vi "Exercise3.vi"() -> ()   [LabVIEW 2016]
uses:
  <vilib>/Utility/file.llb/Write Delimited Spreadsheet (DBL).vi
  Classes/Controller/Motion/Motion Folder/Motion.lvclass
  Classes/Controller/I-O/I-O Folder/I-O.lvclass
  Classes/Controller/Controller Folder/Controller.lvclass
panel:
  in  "file path (dialog if empty)":path=path "D:/Gantry_General/Qualification Results/Exercise3/FInal Combine.txt"
  in  "Final Sensor":path=path "D:/Gantry_General/Qualification Results/Exercise3/Final Sensor.txt"
  out "Bellow position 4":dbl[](array[numeric])=[936.279, 64.123, 66.649, 0.0]
  out "Bellow position 3":dbl[](array[numeric])=[353.0239567258022, 98.85055613080435, 59.0791979543358, 1.5763766432237363]
  out "Bellow position 2":dbl[](array[numeric])=[608.3519774161907, 47.80550407841485, 51.02600004353454, 0.5267134461077569]
  out "Bellow position":dbl[](array[numeric])=[936.279, 64.123, 66.649, 0.0]
  in  "Stop":bool
  in  "Put down pickup tool":bool
  in  "Put down sensor":bool
  in  "Pickup Sensor":bool
  in  "Pickup Pickup Tool":bool
  out "Vacuum OK":bool
  in  "Tray 3":bool
  out "Pickup Tool Center":dbl[](array[numeric])=[1056.142, 74.613, 66.649, 0.0]
  in  "Pickup Tool rotation":dbl=3.14159
  in  "Pickup Tool Path":path=path "D:/Gantry_General/Qualification Results/Exercise3/Pickuptool.txt"
  in  "Sensor":bool
  out "Sensor Center":dbl[](array[numeric])=[728.2149774161908, 58.29550407841485, 51.02600004353454, 0.5267134461077569]
  in  "Sensor rotation":dbl=3.14159
  in  "Sensor Path":path=path "D:/Gantry_General/Qualification Results/Exercise3/Sensor.txt"
  in  "Place position wrt\n Tray Center":dbl[](array[numeric])=[95.0, 0.0, 0.0, 0.0]
  in  "Tray Path":path=path "D:/Gantry_General/Qualification Results/Exercise3/tray.txt"
  in  "Tray rotation":dbl=5.14872
  out "Tray Center":dbl[](array[numeric])=[472.8869567258022, 109.34055613080434, 59.0791979543358, 1.5763766432237363]
  in  "Alignment finish":bool
  in  "Tray":bool
  in  "Final position vacuum":i32=22
  in  "Baseplate mark vacuum":i32=-1
  in  "Sensor Vacuum":i32=20
  in  "Baseplate Region Vacuum":i32=23
  in  "Sensor Regiopn Vacuum":i32=21
  in  "Pickup?":bool=TRUE
  in  "Pickup Go":bool
  # "Gantry Qualification Exercise 3\n1. Place Material"
  # "Alignment settings"
  # "Initialize Vacuum Setup"
  # "( rotation expressed in radians )"
  # "Align material"
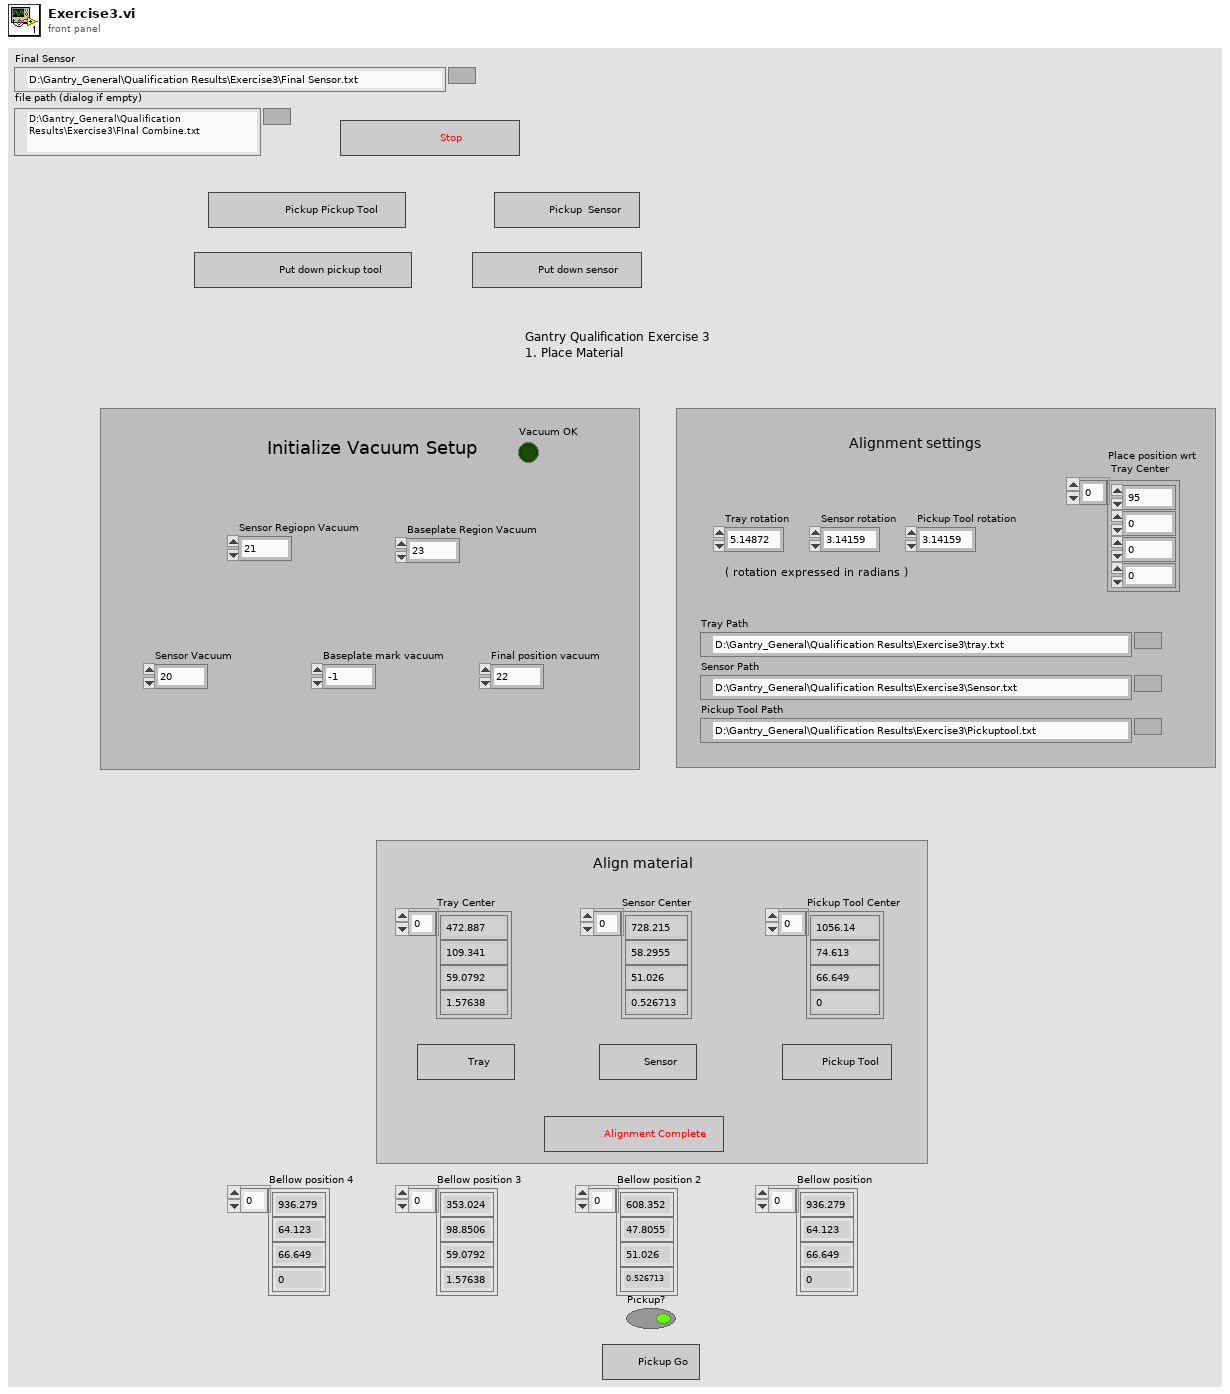
[diagram p1: front panel]
types:
  T1 = typedef "Controller.lvclass/Controllers.ctl" = cluster{"Copy of Motion.lvclass":refnum<class "Motion.lvclass">, "Copy of I-O.lvclass ":refnum<class "I-O.lvclass">, "Copy of Dispenser.lvclass":refnum<class "Dispenser.lvclass">}
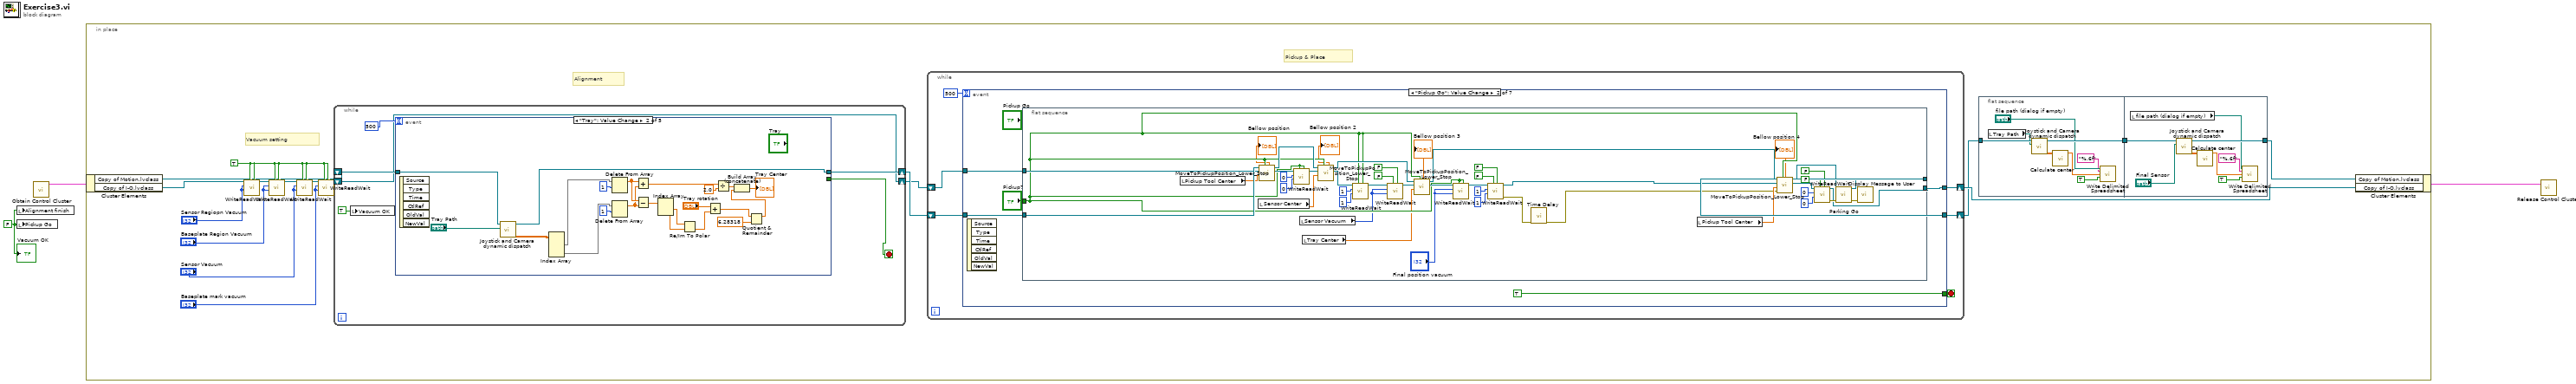
[diagram p0: block diagram]
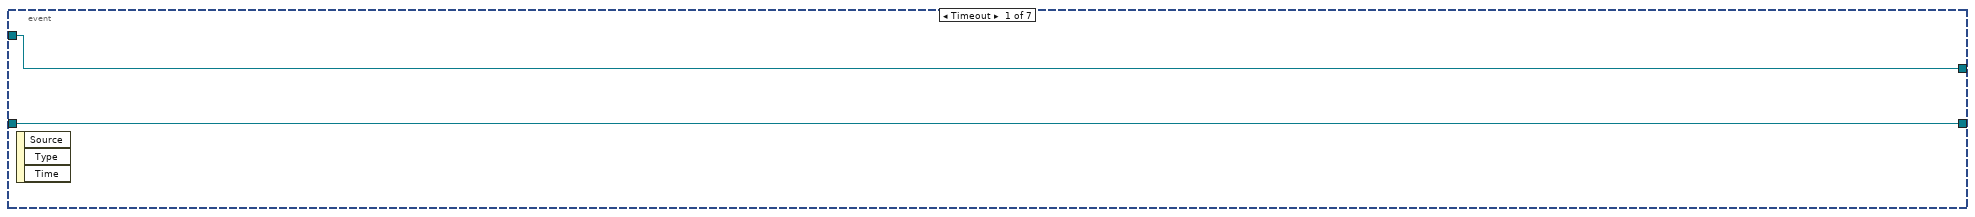
[diagram p2: hidden frame]
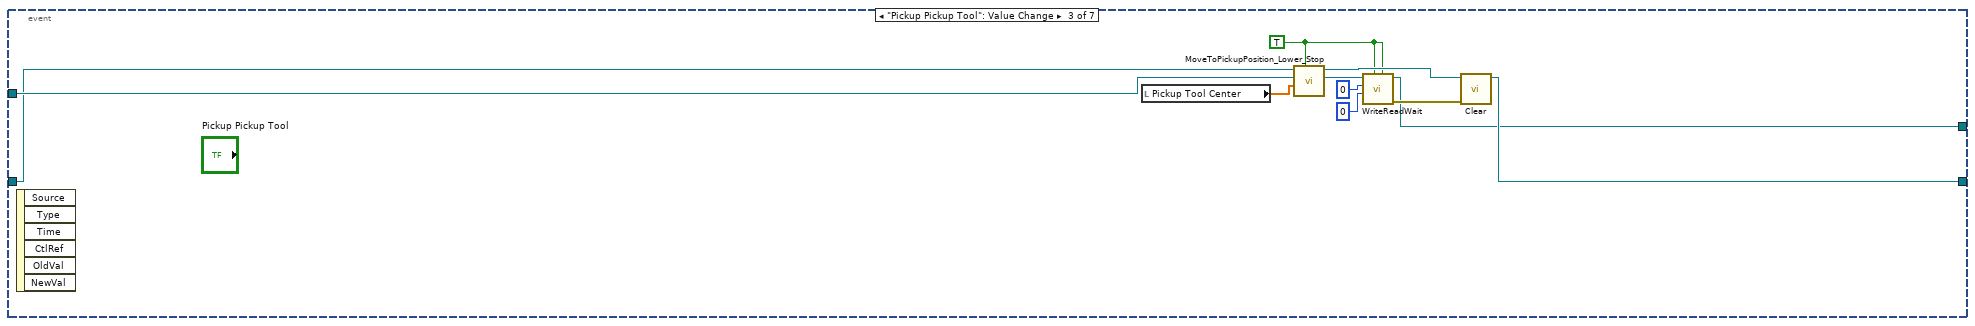
[diagram p3: hidden frame]
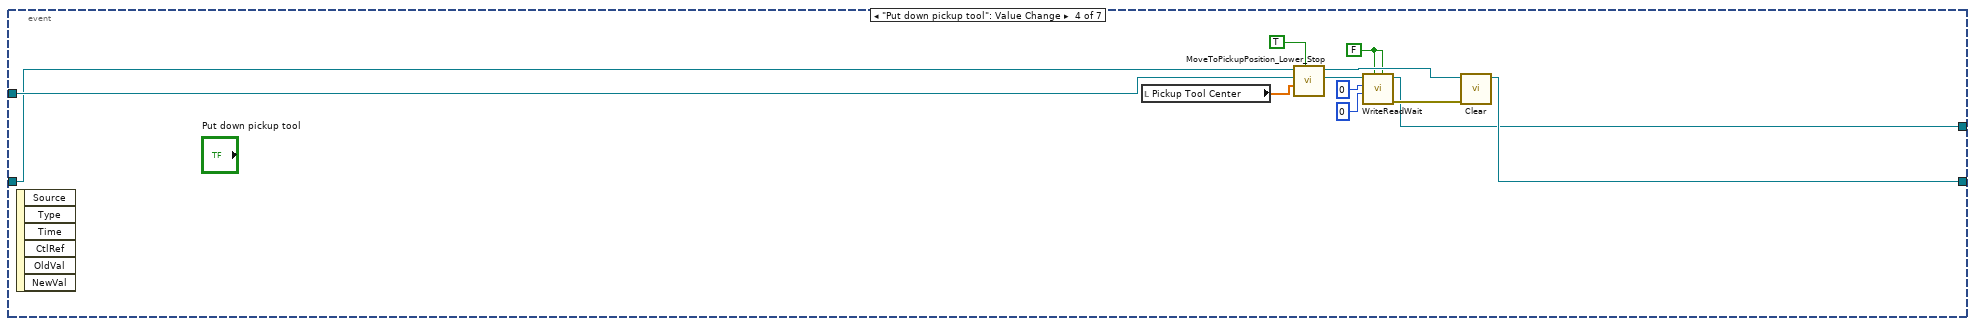
[diagram p4: hidden frame]
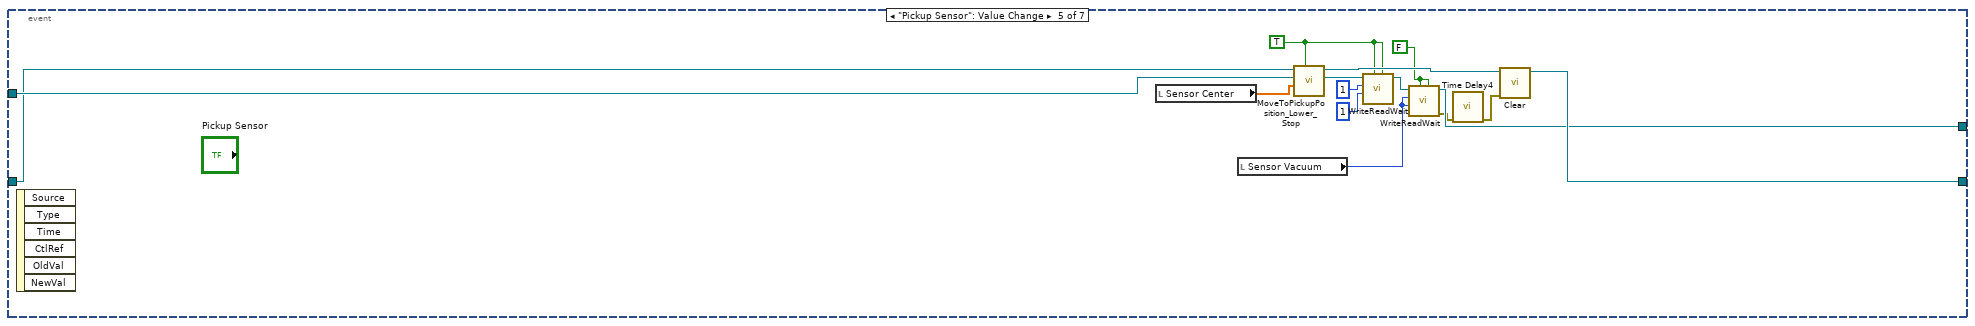
[diagram p5: hidden frame]
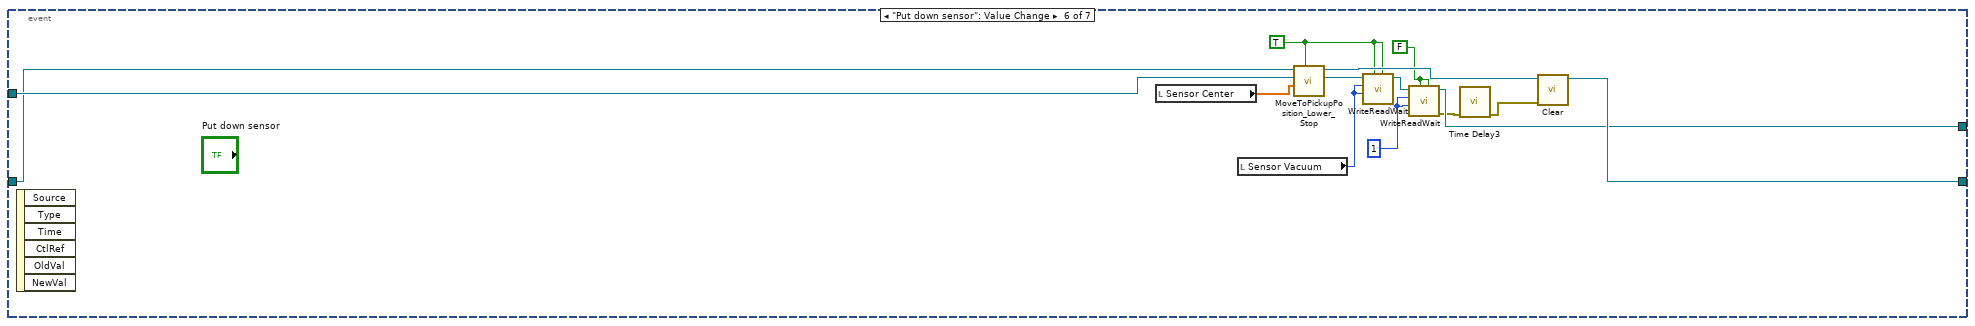
[diagram p6: hidden frame]
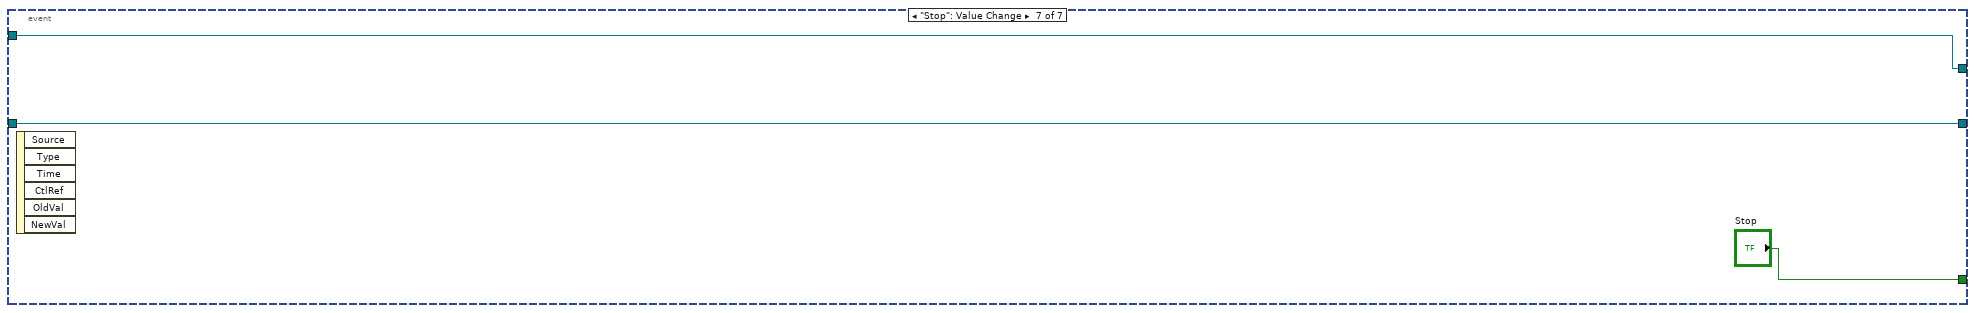
[diagram p7: hidden frame]
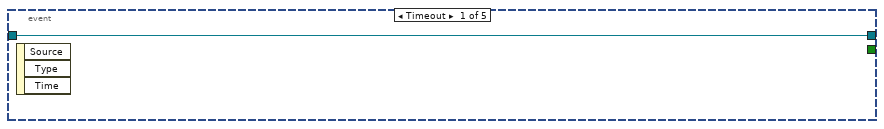
[diagram p8: hidden frame]
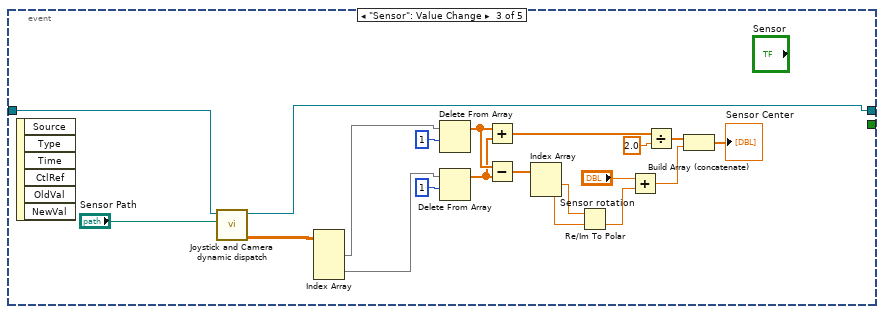
[diagram p9: hidden frame]
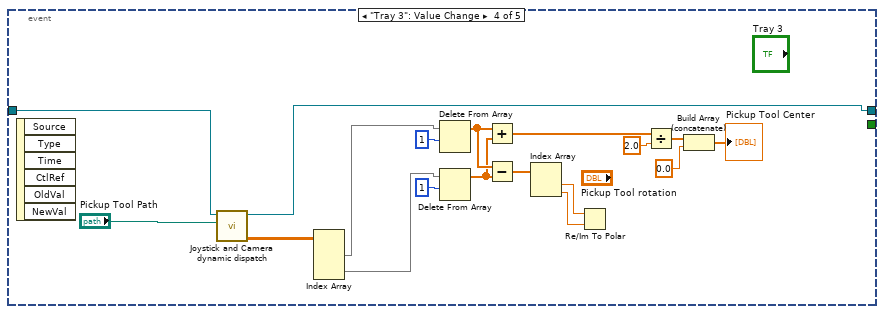
[diagram p10: hidden frame]
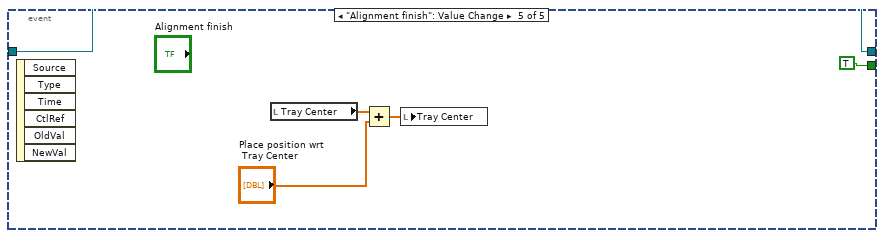
[diagram p11: hidden frame]
diagram:
  w1 = FALSE
  n1 = local write "Alignment finish"(w1) -> ()
  n2 = local write "Pickup Go"(w1) -> ()
  n3 = call "Obtain Control Cluster.vi"() -> ("Control Out"=w3:T1)  [unwired: 11 in]
  n4 = in-place {
    w14 = TRUE ("Read Value")
    # "Vacuum setting"
    # "Pickup & Place"
    # "Alignment"
    n5 = in-place-cluster #1(w3) -> ("Copy of Motion.lvclass"=w11:refnum<class "Motion.lvclass">, "Copy of I-O.lvclass"=w10:refnum<class "I-O.lvclass">)
    n6 = call "WriteReadWait.vi"("Read Value"=w14, "Write Value"=w14, "Read"="Sensor Regiopn Vacuum", "Write"="Sensor Regiopn Vacuum", "I-O in"=w10) -> ("I-O out"=w20:refnum<class "I-O.lvclass">)  [unwired: 5 in, 1 out]
    n7 = call "WriteReadWait.vi"("Read Value"=w14, "Write Value"=w14, "Read"="Baseplate Region Vacuum", "Write"="Baseplate Region Vacuum", "I-O in"=w20) -> ("I-O out"=w19:refnum<class "I-O.lvclass">)  [unwired: 5 in, 1 out]
    n8 = call "WriteReadWait.vi"("Read Value"=w14, "Write Value"=w14, "Read"="Sensor Vacuum", "Write"="Sensor Vacuum", "I-O in"=w19) -> ("I-O out"=w15:refnum<class "I-O.lvclass">)  [unwired: 5 in, 1 out]
    n9 = call "WriteReadWait.vi"("Read Value"=w14, "Write Value"=w14, "Read"="Baseplate mark vacuum", "Write"="Baseplate mark vacuum", "I-O in"=w15) -> ("I-O out"=w8:refnum<class "I-O.lvclass">)  [unwired: 5 in, 1 out]
    n10 = while {
      shift-right: [w155] -> w12
      shift-left: w11 -> [w157]
      shift-right: [w153] -> w7
      shift-left: w8 -> [w153]
      stop <- w156 stop-if-true
      n11 = local write "Vacuum OK"(TRUE ("Vacuum OK")) -> ()
      n12 = event shown="[1] \"Tray\": Value Change" {
        selector: _ -> [_ _ _ _ _]
        dyn-events: _ -> [_ _ _ _ _]
        timeout: 500 -> [_ _ _ _ _]
        tunnel: w157 -> [w158 w180 w200 w218 w222]
        tunnel: [w158 w171 w191 w211 w222] -> w155
        tunnel: [_ _ _ _ TRUE] -> w156
        event Timeout {
          n13 = event-data() -> ()  [unwired: 1 in, 3 out]
        }
        event "Tray": Value Change {
          n14 = event-data() -> ()  [unwired: 1 in, 6 out]
          n15 = call "Joystick and Camera dynamic dispatch.vi"("Tray Path"="Tray Path", "Motion in"=w180) -> ("Fiducial Mark Position"=w170:dbl[][], "Motion out"=w171:refnum<class "Motion.lvclass">)  [unwired: 4 in, 2 out]
          n16 = Index Array(array=w170) -> (element #1=w169:dbl[], element #2=w168:dbl[])  [unwired: 4 in]
          n17 = Delete From Array(array=w169, length=1) -> (array with subset deleted=w167:dbl[])  [unwired: 1 in, 1 out]
          n18 = Delete From Array(array=w168, length=1) -> (array with subset deleted=w166:dbl[])  [unwired: 1 in, 1 out]
          n19 = Add(x=w167, y=w166) -> (x+y=w177:dbl[])
          n20 = Subtract(x=w167, y=w166) -> (x-y=w165:dbl[])
          n21 = Index Array(array=w165) -> (element #1=w164:dbl, element #2=w163:dbl)  [unwired: 2 in]
          n22 = Re/Im To Polar(2:w163, 3:w164) -> (0:w179:dbl)  [unwired: 1 out]
          n23 = Add(x="Tray rotation", y=w179) -> (x+y=w162:dbl)
          n24 = Divide(x=w177, y=2.0) -> (x/y=w178:dbl[])
          n25 = Quotient & Remainder(x=w162, y=6.28318) -> (x-y*floor(x/y)=w159:dbl)  [unwired: 1 out]
          n26 = Build Array (concatenate)(w178, w159) -> (→"Tray Center":dbl[])
        }
        event "Sensor": Value Change {
          n27 = event-data() -> ()  [unwired: 1 in, 6 out]
          n28 = call "Joystick and Camera dynamic dispatch.vi"("Tray Path"="Sensor Path", "Motion in"=w200) -> ("Fiducial Mark Position"=w190:dbl[][], "Motion out"=w191:refnum<class "Motion.lvclass">)  [unwired: 4 in, 2 out]
          n29 = Index Array(array=w190) -> (element #1=w189:dbl[], element #2=w188:dbl[])  [unwired: 4 in]
          n30 = Delete From Array(array=w189, length=1) -> (array with subset deleted=w187:dbl[])  [unwired: 1 in, 1 out]
          n31 = Delete From Array(array=w188, length=1) -> (array with subset deleted=w186:dbl[])  [unwired: 1 in, 1 out]
          n32 = Add(x=w187, y=w186) -> (x+y=w197:dbl[])
          n33 = Subtract(x=w187, y=w186) -> (x-y=w185:dbl[])
          n34 = Index Array(array=w185) -> (element #1=w184:dbl, element #2=w183:dbl)  [unwired: 2 in]
          n35 = Re/Im To Polar(2:w183, 3:w184) -> (0:w199:dbl)  [unwired: 1 out]
          n36 = Add(x="Sensor rotation", y=w199) -> (x+y=w182:dbl)
          n37 = Divide(x=w197, y=2.0) -> (x/y=w198:dbl[])
          n38 = Build Array (concatenate)(w198, w182) -> (→"Sensor Center":dbl[])
        }
        event "Tray 3": Value Change {
          n39 = event-data() -> ()  [unwired: 1 in, 6 out]
          n40 = call "Joystick and Camera dynamic dispatch.vi"("Tray Path"="Pickup Tool Path", "Motion in"=w218) -> ("Fiducial Mark Position"=w210:dbl[][], "Motion out"=w211:refnum<class "Motion.lvclass">)  [unwired: 4 in, 2 out]
          n41 = Index Array(array=w210) -> (element #1=w209:dbl[], element #2=w208:dbl[])  [unwired: 4 in]
          n42 = Delete From Array(array=w209, length=1) -> (array with subset deleted=w207:dbl[])  [unwired: 1 in, 1 out]
          n43 = Delete From Array(array=w208, length=1) -> (array with subset deleted=w206:dbl[])  [unwired: 1 in, 1 out]
          n44 = Add(x=w207, y=w206) -> (x+y=w216:dbl[])
          n45 = Subtract(x=w207, y=w206) -> (x-y=w205:dbl[])
          n46 = Index Array(array=w205) -> (element #1=w204:dbl, element #2=w203:dbl)  [unwired: 2 in]
          n47 = Re/Im To Polar(2:w203, 3:w204) -> ()  [unwired: 2 out]
          n48 = Divide(x=w216, y=2.0) -> (x/y=w217:dbl[])
          n49 = Build Array (concatenate)(w217, 0.0 ("y")) -> (→"Pickup Tool Center":dbl[])
        }
        event "Alignment finish": Value Change {
          n50 = event-data() -> ()  [unwired: 1 in, 6 out]
          n51 = local read "Tray Center"() -> (w221:dbl[])
          n52 = Add(x=w221, y="Place position wrt\n Tray Center") -> (x+y=w220:dbl[])
          n53 = local write "Tray Center"(w220) -> ()
        }
      }
    }
    n54 = while {
      shift-right: [w39] -> w9
      shift-left: w7 -> [w41]
      shift-right: [w38] -> w6
      shift-left: w12 -> [w42]
      stop <- w40 stop-if-true
      n55 = event shown="[1] \"Pickup Go\": Value Change" {
        selector: _ -> [_ _ _ _ _ _ _]
        dyn-events: _ -> [_ _ _ _ _ _ _]
        timeout: 500 -> [_ _ _ _ _ _ _]
        tunnel: w42 -> [w43 w50 w102 w114 w129 w145 w150]
        tunnel: w41 -> [w44 w49 w103 w115 w130 w146 w149]
        tunnel: [_ TRUE _ _ _ _ "Stop"] -> w40
        tunnel: [w44 w45 w98 w110 w124 w140 w149] -> w39
        tunnel: [w43 w46 w99 w111 w127 w143 w150] -> w38
        event Timeout {
          n56 = event-data() -> ()  [unwired: 1 in, 3 out]
        }
        event "Pickup Go": Value Change {
          n57 = event-data() -> ()  [unwired: 1 in, 6 out]
          n58 = flat-sequence {
            tunnel: w50 -> [w84]
            tunnel: w49 -> [w75]
            tunnel: "Pickup?" -> [w63]
            tunnel: [w66] -> w46
            tunnel: [w59] -> w45
            frame #0 {
              n59 = local read "Pickup Tool Center"() -> (w83:dbl[])
              n60 = local read "Sensor Center"() -> (w54:dbl[])
              n61 = call "MoveToPickupPosition_Lower_Stop.vi"("Lower?"=w63, "XYZTheta In"=w83, "I-O in"=w75, "Motion in"=w84) -> ("I-O out"=w82:refnum<class "I-O.lvclass">, "Motion out"=w80:refnum<class "Motion.lvclass">, "Bellow position"=→"Bellow position":dbl[])  [unwired: 4 in, 1 out]
              n62 = call "WriteReadWait.vi"("Read Value"=w63, "Write Value"=w63, "Read"=0, "Write"=0, "I-O in"=w82) -> ("I-O out"=w81:refnum<class "I-O.lvclass">)  [unwired: 5 in, 1 out]
              n63 = local read "Sensor Vacuum"() -> (w53:i32)
              n64 = local read "Tray Center"() -> (w52:dbl[])
              n65 = call "MoveToPickupPosition_Lower_Stop.vi"("Lower?"=w63, "XYZTheta In"=w54, "I-O in"=w81, "Motion in"=w80) -> ("I-O out"=w79:refnum<class "I-O.lvclass">, "Motion out"=w78:refnum<class "Motion.lvclass">, "Bellow position"=→"Bellow position 2":dbl[])  [unwired: 4 in, 1 out]
              n66 = call "WriteReadWait.vi"("Read Value"=w63, "Write Value"=w63, "Read"=1, "Write"=1, "I-O in"=w79) -> ("I-O out"=w90:refnum<class "I-O.lvclass">)  [unwired: 5 in, 1 out]
              n67 = call "WriteReadWait.vi"("Read Value"=FALSE, "Write Value"=FALSE, "Read"=w53, "Write"=w53, "I-O in"=w90) -> ("I-O out"=w77:refnum<class "I-O.lvclass">)  [unwired: 5 in, 1 out]
              n68 = call "MoveToPickupPosition_Lower_Stop.vi"("Lower?"=w63, "XYZTheta In"=w52, "I-O in"=w77, "Motion in"=w78) -> ("I-O out"=w76:refnum<class "I-O.lvclass">, "Motion out"=w61:refnum<class "Motion.lvclass">, "Bellow position"=→"Bellow position 3":dbl[])  [unwired: 4 in, 1 out]
              n69 = call "WriteReadWait.vi"("Read Value"=w63, "Write Value"=w63, "Read"="Final position vacuum", "Write"="Final position vacuum", "I-O in"=w76) -> ("I-O out"=w85:refnum<class "I-O.lvclass">)  [unwired: 5 in, 1 out]
              n70 = call "WriteReadWait.vi"("Read Value"=FALSE, "Write Value"=FALSE, "Read"=1, "Write"=1, "I-O in"=w85) -> ("error out"=w64:errorcluster, "I-O out"=w60:refnum<class "I-O.lvclass">)  [unwired: 5 in]
              n71 = call "Time Delay"("error in (no error)"=w64) -> ("error out"=w62:errorcluster)  [unwired: 10 in]
              n72 = local read "Pickup Tool Center"() -> (w74:dbl[])
              n73 = call "MoveToPickupPosition_Lower_Stop.vi"("Lower?"=w63, "error in (no error)"=w62, "XYZTheta In"=w74, "I-O in"=w60, "Motion in"=w61) -> ("I-O out"=w73:refnum<class "I-O.lvclass">, "Motion out"=w68:refnum<class "Motion.lvclass">, "Bellow position"=→"Bellow position 4":dbl[])  [unwired: 3 in, 1 out]
              n74 = call "WriteReadWait.vi"("Read Value"=FALSE, "Write Value"=FALSE, "Read"=0, "Write"=0, "I-O in"=w73) -> ("error out"=w67:errorcluster, "I-O out"=w59:refnum<class "I-O.lvclass">)  [unwired: 5 in]
              n75 = call-dynamic "Parking Go.vi"("error in (no error)"=w67, "Motion in"=w68) -> ("error out"=w65:errorcluster, "Motion out"=w66:refnum<class "Motion.lvclass">)  [unwired: 8 in]
              n76 = call "Display Message to User"("error in (no error)"=w65) -> ()  [unwired: 9 in, 2 out]
            }
          }
        }
        event "Pickup Pickup Tool": Value Change {
          w97 = TRUE ("Lower?")
          n77 = event-data() -> ()  [unwired: 1 in, 6 out]
          n78 = local read "Pickup Tool Center"() -> (w105:dbl[])
          n79 = call "MoveToPickupPosition_Lower_Stop.vi"("Lower?"=w97, "XYZTheta In"=w105, "I-O in"=w103, "Motion in"=w102) -> ("I-O out"=w104:refnum<class "I-O.lvclass">, "Motion out"=w101:refnum<class "Motion.lvclass">)  [unwired: 4 in, 2 out]
          n80 = call "WriteReadWait.vi"("Read Value"=w97, "Write Value"=w97, "Read"=0, "Write"=0, "I-O in"=w104) -> ("error out"=w100:errorcluster, "I-O out"=w98:refnum<class "I-O.lvclass">)  [unwired: 5 in]
          n81 = call "Clear.vi"("error in (no error)"=w100, "Motion in"=w101) -> ("Motion out"=w99:refnum<class "Motion.lvclass">)  [unwired: 8 in, 1 out]
        }
        event "Put down pickup tool": Value Change {
          w108 = FALSE ("Read Value")
          n82 = event-data() -> ()  [unwired: 1 in, 6 out]
          n83 = local read "Pickup Tool Center"() -> (w117:dbl[])
          n84 = call "MoveToPickupPosition_Lower_Stop.vi"("Lower?"=TRUE, "XYZTheta In"=w117, "I-O in"=w115, "Motion in"=w114) -> ("I-O out"=w116:refnum<class "I-O.lvclass">, "Motion out"=w113:refnum<class "Motion.lvclass">)  [unwired: 4 in, 2 out]
          n85 = call "WriteReadWait.vi"("Read Value"=w108, "Write Value"=w108, "Read"=0, "Write"=0, "I-O in"=w116) -> ("error out"=w112:errorcluster, "I-O out"=w110:refnum<class "I-O.lvclass">)  [unwired: 5 in]
          n86 = call "Clear.vi"("error in (no error)"=w112, "Motion in"=w113) -> ("Motion out"=w111:refnum<class "Motion.lvclass">)  [unwired: 8 in, 1 out]
        }
        event "Pickup Sensor": Value Change {
          w122 = FALSE ("Read Value")
          w126 = TRUE ("Lower?")
          n87 = event-data() -> ()  [unwired: 1 in, 6 out]
          n88 = local read "Sensor Center"() -> (w132:dbl[])
          n89 = local read "Sensor Vacuum"() -> (w123:i32)
          n90 = call "MoveToPickupPosition_Lower_Stop.vi"("Lower?"=w126, "XYZTheta In"=w132, "I-O in"=w130, "Motion in"=w129) -> ("I-O out"=w131:refnum<class "I-O.lvclass">, "Motion out"=w128:refnum<class "Motion.lvclass">)  [unwired: 4 in, 2 out]
          n91 = call "WriteReadWait.vi"("Read Value"=w126, "Write Value"=w126, "Read"=1, "Write"=1, "I-O in"=w131) -> ("I-O out"=w125:refnum<class "I-O.lvclass">)  [unwired: 5 in, 1 out]
          n92 = call "WriteReadWait.vi"("Read Value"=w122, "Write Value"=w122, "Read"=w123, "Write"=w123, "I-O in"=w125) -> ("error out"=w121:errorcluster, "I-O out"=w124:refnum<class "I-O.lvclass">)  [unwired: 5 in]
          n93 = call "Time Delay4"("error in (no error)"=w121) -> ("error out"=w120:errorcluster)  [unwired: 10 in]
          n94 = call "Clear.vi"("error in (no error)"=w120, "Motion in"=w128) -> ("Motion out"=w127:refnum<class "Motion.lvclass">)  [unwired: 8 in, 1 out]
        }
        event "Put down sensor": Value Change {
          w137 = 1 ("Write")
          w139 = FALSE ("Read Value")
          w142 = TRUE ("Lower?")
          n95 = event-data() -> ()  [unwired: 1 in, 6 out]
          n96 = local read "Sensor Center"() -> (w148:dbl[])
          n97 = local read "Sensor Vacuum"() -> (w138:i32)
          n98 = call "MoveToPickupPosition_Lower_Stop.vi"("Lower?"=w142, "XYZTheta In"=w148, "I-O in"=w146, "Motion in"=w145) -> ("I-O out"=w147:refnum<class "I-O.lvclass">, "Motion out"=w144:refnum<class "Motion.lvclass">)  [unwired: 4 in, 2 out]
          n99 = call "WriteReadWait.vi"("Read Value"=w142, "Write Value"=w142, "Read"=w138, "Write"=w138, "I-O in"=w147) -> ("I-O out"=w141:refnum<class "I-O.lvclass">)  [unwired: 5 in, 1 out]
          n100 = call "WriteReadWait.vi"("Read Value"=w139, "Write Value"=w139, "Read"=w137, "Write"=w137, "I-O in"=w141) -> ("error out"=w136:errorcluster, "I-O out"=w140:refnum<class "I-O.lvclass">)  [unwired: 5 in]
          n101 = call "Time Delay3"("error in (no error)"=w136) -> ("error out"=w135:errorcluster)  [unwired: 10 in]
          n102 = call "Clear.vi"("error in (no error)"=w135, "Motion in"=w144) -> ("Motion out"=w143:refnum<class "Motion.lvclass">)  [unwired: 8 in, 1 out]
        }
        event "Stop": Value Change {
          n103 = event-data() -> ()  [unwired: 1 in, 6 out]
        }
      }
    }
    n104 = flat-sequence {
      tunnel: w6 -> [w28]
      tunnel: [w26] -> w5
      tunnel: w5 -> [w35]
      tunnel: [w34] -> w4
      frame #0 {
        n105 = local read "Tray Path"() -> (w27:path)
        n106 = call "Joystick and Camera dynamic dispatch.vi"("Tray Path"=w27, "Motion in"=w28) -> ("Fiducial Mark Position"=w25:dbl[][], "Motion out"=w26:refnum<class "Motion.lvclass">)  [unwired: 4 in, 2 out]
        n107 = call "Calculate center.vi"("array"=w25) -> ("Tray Center"=w24:dbl[])  [unwired: 10 in]
        n108 = call-poly <vilib>:"Write Delimited Spreadsheet.vi"("file path (dialog if empty)"="file path (dialog if empty)", "format (%.3f)"="%.6f", "1D data"=w24, "append to file? (new file:F)"=TRUE) -> ()  [unwired: 10 in, 2 out]
      }
      frame #1 {
        n109 = local read "file path (dialog if empty)"() -> (w29:path)
        n110 = call "Joystick and Camera dynamic dispatch.vi"("Tray Path"="Final Sensor", "Motion in"=w35) -> ("Fiducial Mark Position"=w33:dbl[][], "Motion out"=w34:refnum<class "Motion.lvclass">)  [unwired: 4 in, 2 out]
        n111 = call "Calculate center.vi"("array"=w33) -> ("Tray Center"=w32:dbl[])  [unwired: 10 in]
        n112 = call-poly <vilib>:"Write Delimited Spreadsheet.vi"("file path (dialog if empty)"=w29, "format (%.3f)"="%.6f", "1D data"=w32, "append to file? (new file:F)"=TRUE) -> ()  [unwired: 10 in, 2 out]
      }
    }
    n113 = in-place-cluster #1("Copy of Motion.lvclass"=w4, "Copy of I-O.lvclass"=w9) -> (w2:T1)
  }
  n114 = call "Release Control Cluster.vi"("output cluster"=w2) -> ()  [unwired: 11 in]
  "Vacuum OK" <- w1
